vi "Post_Pro_Results_Hierarchy.vi"() -> ()   [LabVIEW 2016]
uses:
  Anemometry Sub Vis/Globals/Plug_in_data_global.vi
panel:
  in  "Per Block Plug Ins Extra":string[](array[string])
  in  "Template":path
  out "Current File Number":i32
  out "Number of Files to Process":i32
  out "Currently Processing":path
  out "Files to Post Process":path[](array[path])
  in  "Save results to":T1(ring)=enum."Original Results Filenames with _PP"
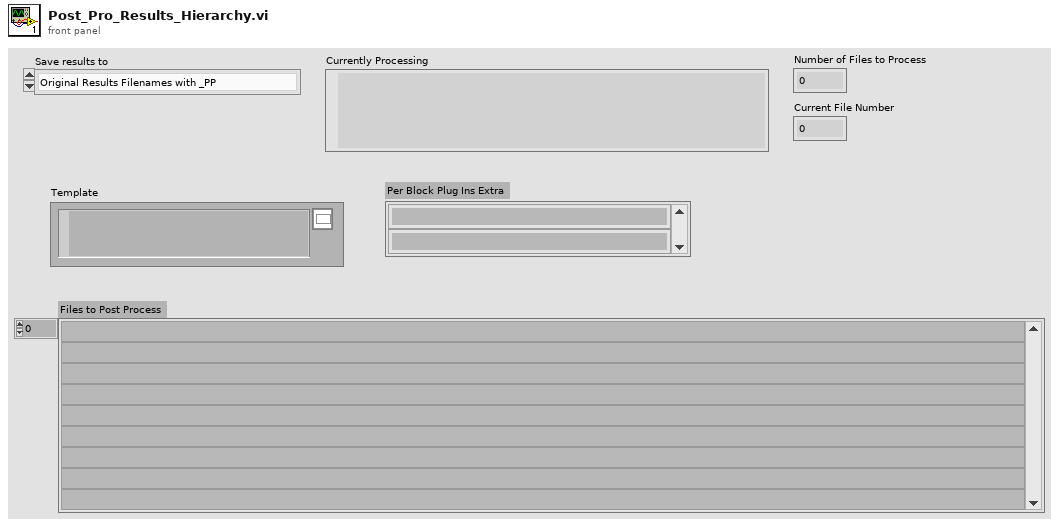
[diagram p1: front panel]
types:
  T1 = enum16{"A single file", "Original Results Filenames with _PP", "Current Results Filenames"}
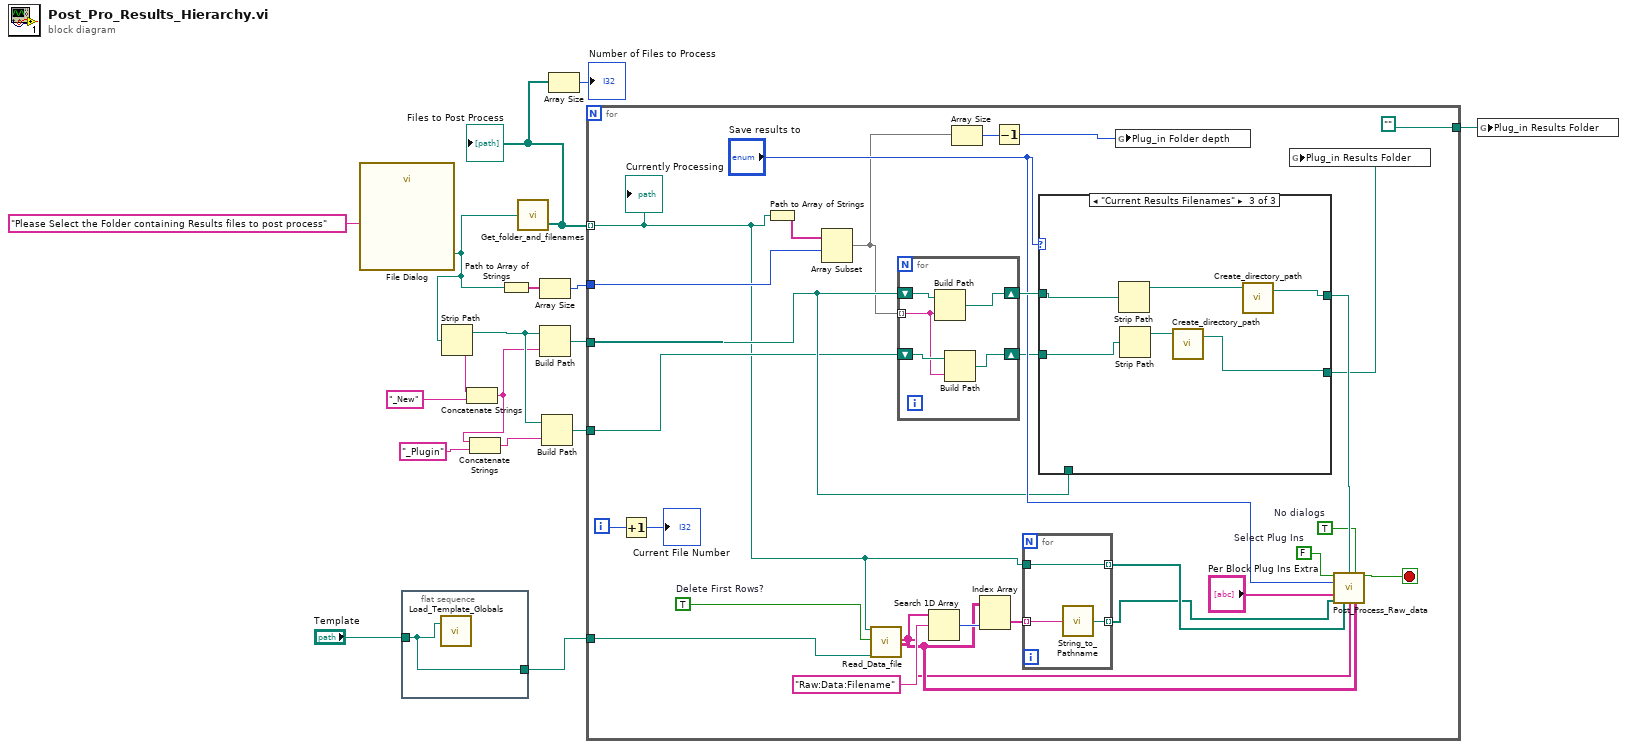
[diagram p0: block diagram]
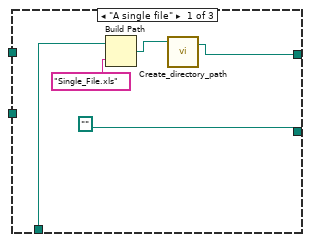
[diagram p2: hidden frame]
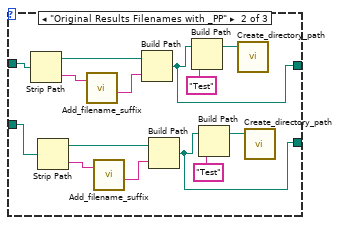
[diagram p3: hidden frame]
diagram:
  n1 = call "File Dialog"("prompt"="Please Select the Folder containing Results files to post process") -> ("selected path"=w14:path)  [unwired: 11 in, 3 out]
  n2 = flat-sequence {
    tunnel: "Template" -> [w18]
    tunnel: [w18] -> w1
    frame #0 {
      n3 = call "Load_Template_Globals.vi"("Template-read"=w18) -> ()  [unwired: 1 in, 1 out]
    }
  }
  n4 = Strip Path(path=w14) -> (stripped path=w8:path, name=w13:string)
  n5 = Concatenate Strings(w13, "_New" ("string")) -> (w7:string)
  n6 = Concatenate Strings(w7, "_Plugin" ("string")) -> (w5:string)
  n7 = Path to Array of Strings(0:w14) -> (2:w16:string[])  [unwired: 1 out]
  n8 = call "Get_folder_and_filenames.vi"("file path (dialog if empty)"=w14) -> ("Files"=w10:path[])  [unwired: 1 out]
  "Files to Post Process" <- w10
  n9 = Array Size(array=w16) -> (size(s)=w15:i32)
  n10 = Build Path(base path=w8, name or relative path=w7) -> (appended path=w11:path)
  n11 = Build Path(base path=w8, name or relative path=w5) -> (appended path=w4:path)
  n12 = Array Size(array=w10) -> (size(s)=→"Number of Files to Process":i32)
  n13 = for {
    tunnel: w10 -> [w32] mode=indexing
    tunnel: w15 -> [w46]
    tunnel: w11 -> [w43]
    tunnel: w4 -> [w39]
    tunnel: w1 -> [w22]
    tunnel: [path ""] -> w3
    i -> [w41]
    stop <- w23 stop-if-true
    w25 = TRUE  # No dialogs
    w26 = FALSE  # Select Plug Ins
    w33 = TRUE  # Delete First Rows?
    n14 = Increment(x=w41) -> (x+1=→"Current File Number":i32)
    n15 = Path to Array of Strings(0:w32) -> (2:w47:string[])  [unwired: 1 out]
    n16 = Array Subset(array=w47, index=w46) -> (w21:string[])  [unwired: 1 in]
    n17 = call "Read_Data_file.vi"("Results file"=w32, "Delete First Rows?"=w33, "Template File"=w22) -> ("Ch names Out"=w27:string[], "Channel Values Out"=w28:string[][])  [unwired: 4 in, 11 out]
    n18 = for {
      tunnel: w21 -> [w76] mode=indexing
      shift-right: [w79] -> w45
      shift-left: w43 -> [w80]
      shift-right: [w78] -> w37
      shift-left: w39 -> [w77]
      n19 = Build Path(base path=w80, name or relative path=w76) -> (appended path=w79:path)
      n20 = Build Path(base path=w77, name or relative path=w76) -> (appended path=w78:path)
    }
    n21 = Search 1D Array(1D array=w27, element="Raw:Data:Filename") -> (index of element=w35:i32)  [unwired: 1 in]
    n22 = Array Size(array=w21) -> (size(s)=w20:i32)
    n23 = Index Array(array=w28, index (col)=w35) -> (element=w36:string[])  [unwired: 1 in]
    n24 = Decrement(x=w20) -> (x-1=w19:i32)
    n25 = for {
      tunnel: w36 -> [w50] mode=indexing
      tunnel: [w49] -> w30 mode=indexing
      tunnel: [w48] -> w31 mode=indexing
      tunnel: w32 -> [w48]
      n26 = call "String_to_Pathname.vi"("Input String"=w50) -> ("path"=w49:path)
    }
    n27 = case shown="\"Current Results Filenames\"" "Save results to" {
      tunnel: w45 -> [_ w68 w74]
      tunnel: [w52 w63 w75] -> w42
      tunnel: w43 -> [w55 _ _]
      tunnel: [path "" w56 w70] -> w38
      tunnel: w37 -> [_ w57 w71]
      frame "A single file" {
        n28 = Build Path(base path=w55, name or relative path="Single_File.xls") -> (appended path=w53:path)
        n29 = call "Create_directory_path.vi"("Path name"=w53) -> ("Path name Out"=w52:path)  [unwired: 2 in, 1 out]
      }
      frame "Original Results Filenames with _PP" {
        n30 = Strip Path(path=w68) -> (stripped path=w66:path, name=w67:string)
        n31 = Strip Path(path=w57) -> (stripped path=w60:path, name=w59:string)
        n32 = call "Add_filename_suffix.vi"("Filename"=w67) -> ("Base name"=w69:string)  [unwired: 1 in, 3 out]
        n33 = call "Add_filename_suffix.vi"("Filename"=w59) -> ("Base name"=w58:string)  [unwired: 1 in, 3 out]
        n34 = Build Path(base path=w66, name or relative path=w69) -> (appended path=w63:path)
        n35 = Build Path(base path=w60, name or relative path=w58) -> (appended path=w56:path)
        n36 = Build Path(base path=w63, name or relative path="Test") -> (appended path=w64:path)
        n37 = Build Path(base path=w56, name or relative path="Test") -> (appended path=w62:path)
        n38 = call "Create_directory_path.vi"("Path name"=w64) -> ()  [unwired: 2 in, 2 out]
        n39 = call "Create_directory_path.vi"("Path name"=w62) -> ()  [unwired: 2 in, 2 out]
      }
      frame "Current Results Filenames" {
        n40 = Strip Path(path=w74) -> (stripped path=w73:path)  [unwired: 1 out]
        n41 = Strip Path(path=w71) -> (stripped path=w72:path)  [unwired: 1 out]
        n42 = call "Create_directory_path.vi"("Path name"=w72) -> ("Path name Out"=w70:path)  [unwired: 2 in, 1 out]
        n43 = call "Create_directory_path.vi"("Path name"=w73) -> ("Path name Out"=w75:path)  [unwired: 2 in, 1 out]
      }
    }
    n44 = global write "Plug_in_data_global.vi" "Plug_in Folder depth"(w19) -> ()
    n45 = global write "Plug_in_data_global.vi" "Plug_in Results Folder"(w38) -> ()
    n46 = call "Post_Process_Raw_data.vi"("Select Plug Ins"=w26, "Post processed Results folder"=w42, "No dialogs"=w25, "Save results to"="Save results to", "Per Block Plug Ins Extra"="Per Block Plug Ins Extra", "Selected files"=w30, "Current Results filenames"=w31, "Results Plotter Channel names"=w27, "Results Plotter Data"=w28) -> ("Stopped"=w23:bool)  [unwired: 5 in, 1 out]
    "Currently Processing" <- w32
  }
  n47 = global write "Plug_in_data_global.vi" "Plug_in Results Folder"(w3) -> ()
